vi "ACIR.vi"(6 "Setting":T1={"Freq"=1000.0, "Range"=enum."10m Ohm", "Measurements"=enum."Impedence"} {"Freq" min=0.1 max=1050.0 step=0.01 format="%_5e"}, 8 "error in":errorcluster, 9 "ACIR Ref":string, 10 "ACIR ClassName":string="Hioki BT4560B.lvclass", 11 "Base Path":path=path "C:/GitHub/OOP_OPC UA/Sequence/CodeModules/HAL/Concrete") -> (0 "error out":errorcluster={"status"=TRUE, "code"=-1073807346, "source"="VISA Open in APS-7000 Series.lvlib:Initialize.vi->Concrete.lvlib:APS7050.lvclass:Initialise.vi->Check objects.vi"}, 3 "Measurements":dbl)   [LabVIEW 2021]
uses:
  HAL/Harware Abstraction/ACIR/ACIR.lvclass
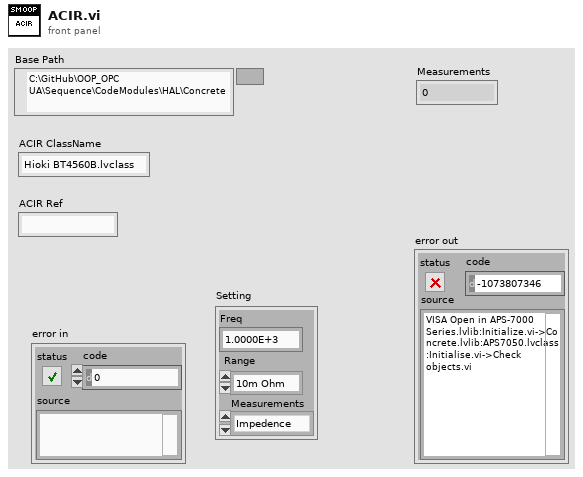
[diagram p1: front panel]
types:
  T1 = cluster{"Freq":dbl, "Range":enum16{"3m Ohm", "10m Ohm", "100m Ohm"}, "Measurements":enum16{"Impedence", "Phase Angle", "OCV"}}
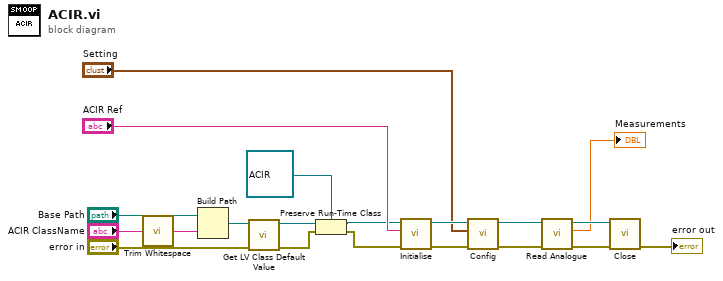
[diagram p0: block diagram]
diagram:
  n1 = call <vilib>:"Trim Whitespace.vi"("string"="ACIR ClassName") -> ("trimmed string"=w18:string)  [unwired: 1 in]
  n2 = Build Path(base path="Base Path", name or relative path=w18) -> (appended path=w16:path)
  n3 = call <vilib>:"Get LV Class Default Value.vi"("error in (no error)"="error in", "class path"=w16) -> ("error out"=w15:errorcluster, "object"=w19:refnum<class>)  [unwired: 8 in]
  n4 = Preserve Run-Time Class(object in=w19, error in=w15, 2:refnum<class "ACIR.lvclass"> refnum ("HAL.lvlib:ACIR.lvclass")) -> (object out=w13:refnum<class "ACIR.lvclass">, error out=w12:errorcluster)
  n5 = call-dynamic "Initialise.vi"("error in (no error)"=w12, "Instrument Ref"="ACIR Ref", "Instrument in"=w13) -> ("error out"=w7:errorcluster, "Instrument out"=w8:refnum<class "ACIR.lvclass">)  [unwired: 7 in]
  n6 = call-dynamic "Config.vi"("error in (no error)"=w7, "Setting"="Setting", "ACIR in"=w8) -> ("error out"=w6:errorcluster, "ACIR out"=w5:refnum<class "ACIR.lvclass">)  [unwired: 7 in]
  n7 = call-dynamic "Read Analogue.vi"("error in (no error)"=w6, "PS in"=w5) -> ("error out"=w4:errorcluster, "Measurements"=→"Measurements":dbl, "PS out"=w3:refnum<class "ACIR.lvclass">)  [unwired: 7 in]
  n8 = call-dynamic "Close.vi"("error in (no error)"=w4, "Instrument in"=w3) -> ("error out"=→"error out":errorcluster)  [unwired: 8 in, 1 out]
